vi "PathPlanner_PathFinder_NewSub1.vi"   [LabVIEW 2019]
uses:
  PathPlannerLib24/VI/PathPlanner_PathFinder_Globals.vi
  PathPlannerLib24/PathPlanner24.lvlib
types:
  T1 = typedef "PathPlanner24.lvlib/PathPlannerFinderDoublePair.ctl" = cluster{"A":dbl, "B":dbl}
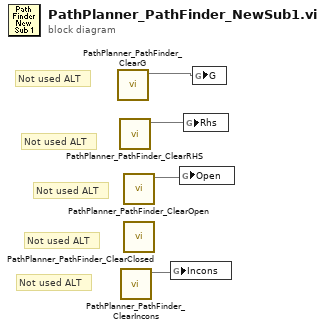
[diagram p0: block diagram]
diagram:
  # "Not used ALT"
  # "Not used ALT"
  # "Not used ALT"
  # "Not used ALT"
  # "Not used ALT"
  n1 = call "PathPlanner_PathFinder_ClearG.vi"() -> ("G"=w3:map{i32, dbl})  [unwired: 11 in]
  n2 = call "PathPlanner_PathFinder_ClearRHS.vi"() -> ("Rhs"=w2:map{i32, dbl})  [unwired: 11 in]
  n3 = call "PathPlanner_PathFinder_ClearIncons.vi"() -> ("Incons"=w4:map{i32, T1})  [unwired: 11 in]
  n4 = call "PathPlanner_PathFinder_ClearOpen.vi"() -> ("Open"=w1:map{i32, T1})  [unwired: 11 in]
  n5 = call "PathPlanner_PathFinder_ClearClosed.vi"() -> ()  [unwired: 11 in, 1 out]
  n6 = global write "PathPlanner_PathFinder_Globals.vi" "Incons"(w4) -> ()
  n7 = global write "PathPlanner_PathFinder_Globals.vi" "Open"(w1) -> ()
  n8 = global write "PathPlanner_PathFinder_Globals.vi" "Rhs"(w2) -> ()
  n9 = global write "PathPlanner_PathFinder_Globals.vi" "G"(w3) -> ()
